vi "Send Stop Event MessengerM.vi"(7 "subchannel":i32, 8 "sync in":errorcluster) -> (2 "channel":T1)   [LabVIEW 2025]
uses:
  <extravilib>/ChannelInstances/Event Messenger-c(str,var)/))Channel.vi
  Event-MessengerM-Channel-Wire/source/Event MessengerM.lvlib
  Event-MessengerM-Channel-Wire/source/))Channel.ctl
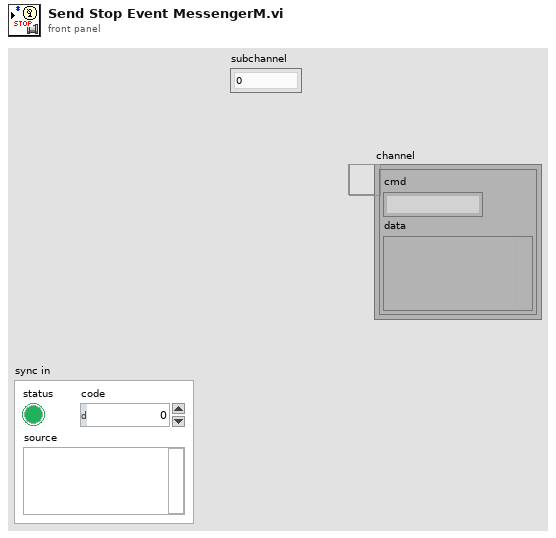
[diagram p1: front panel]
types:
  T1 = typedef "Event MessengerM.lvlib/))Channel.ctl" = refnum<queue>
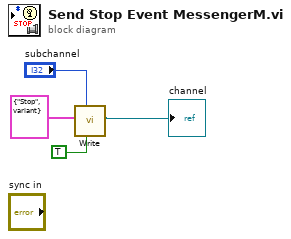
[diagram p0: block diagram]
diagram:
  n1 = call "Write.vi"("high priority? (F)"=TRUE, "subchannel (0)"="subchannel", "element"=cluster{"cmd":string, "data":variant} {"cmd"="Stop", "data"=variant} ("message")) -> ("channel"=→"channel":T1)  [unwired: 7 in, 1 out]
